vi "Remove All.vi"(8 "error in (no error)":errorcluster, 10 "Action":T1, 11 "Custom Device reference in":refnum<k24>) -> (0 "error out":errorcluster, 3 "Custom Device reference out":refnum<k24>)   [LabVIEW 2019, in "J1939 System Definition API Support.lvlib"]
uses:
  J1939 System Definition API Support.lvlib
  NationalInstruments.VeriStand.SystemDefinitionAPI
  <vilib>/NI VeriStand/Custom Device Tools/Custom Device Utility Library/Custom Device Utility Library.lvlib
  Shared/SubVIs/Constants.vi
  Shared/J1939 Addon Shared.lvlib
  <vilib>/NI VeriStand/Custom Device API/Custom Device API.lvlib
  <vilib>/NI VeriStand/Custom Device Tools/Custom Device Utility Library/NI VeriStand - Search for All Items by GUID.vi
  Types/Remove Frame Action.ctl
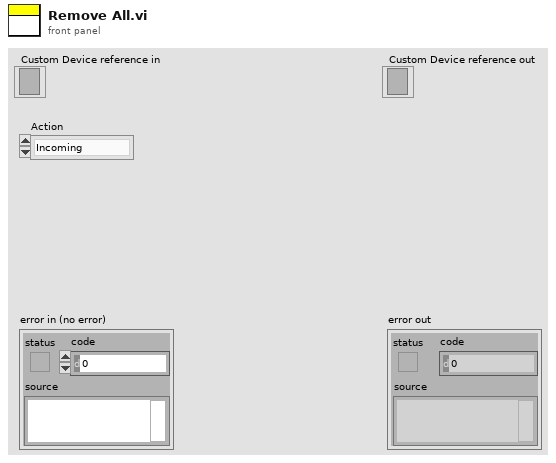
[diagram p1: front panel]
types:
  T1 = typedef "J1939 System Definition API Support.lvlib/Remove Frame Action.ctl" = enum16{"Incoming", "Outgoing Event", "Outgoing Cyclic", "Outgoing Cyclic Event"}
  T2 = typedef "Custom Device API.lvlib/Custom Device Item Ref.ctl" = u64
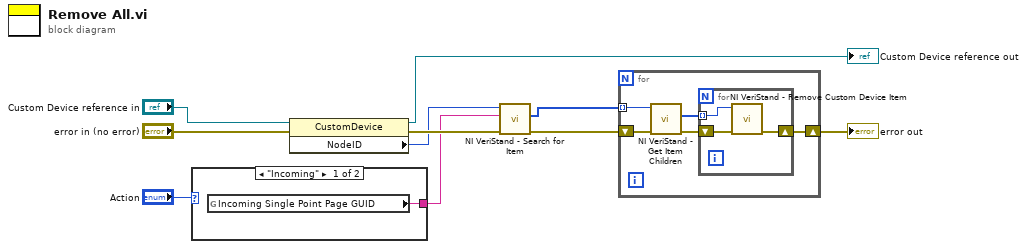
[diagram p0: block diagram]
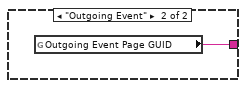
[diagram p2: hidden frame]
diagram:
  n1 = case shown="\"Incoming\"" "Action" {
    tunnel: [w11 w12] -> w6
    frame "Incoming" {
      n2 = global read "Constants.vi" "Incoming Single Point Page GUID"() -> (w11:string)
    }
    frame "Outgoing Event" {
      n3 = global read "Constants.vi" "Outgoing Event Page GUID"() -> (w12:string)
    }
  }
  n4 = property class="CustomDevice"(reference="Custom Device reference in", error in="error in (no error)") -> (reference out=→"Custom Device reference out":refnum<k24>, error out=w7:errorcluster, "NodeID"=w5:u64)
  n5 = call-poly <vilib>:"NI VeriStand - Search for Item.vi"("error in"=w7, "Item GUID"=w6, "Section Ref in"=w5) -> ("error out"=w1:errorcluster, "Item Refs"=w2:T2[])  [unwired: 5 in, 2 out]
  n6 = for {
    tunnel: w2 -> [w16] mode=indexing
    shift-right: [w17] -> w4
    shift-left: w1 -> [w14]
    n7 = call <vilib>:"NI VeriStand - Get Item Children.vi"("error in (no error)"=w14, "Item Ref in"=w16) -> ("error out"=w13:errorcluster, "Child Refs"=w15:T2[])  [unwired: 6 in, 2 out]
    n8 = for {
      tunnel: w15 -> [w18] mode=indexing
      shift-right: [w20] -> w17
      shift-left: w13 -> [w19]
      n9 = call <vilib>:"NI VeriStand - Remove Custom Device Item.vi"("error in (no error)"=w19, "Item Ref in"=w18) -> ("error out"=w20:errorcluster)  [unwired: 8 in, 1 out]
    }
  }
  "error out" <- w4
